vi "X calculator.vi"(9 "Blue":i16, 10 "Green":i16, 11 "Red":i16) -> (3 "X":dbl)   [LabVIEW 2014, in "AMS TS3472 Light Sensor.lvlib" / "AMS TCS3472.lvclass"]
uses:
  AMS TCS3472.lvclass
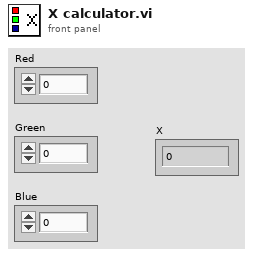
[diagram p1: front panel]
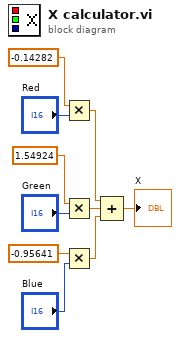
[diagram p0: block diagram]
diagram:
  n1 = Multiply(x=-0.14282, y="Red") -> (x*y=w7:dbl)
  n2 = Multiply(x=1.54924, y="Green") -> (x*y=w6:dbl)
  n3 = Multiply(x=-0.95641, y="Blue") -> (x*y=w5:dbl)
  n4 = Compound Arithmetic op=ADD(w7, w6, w5) -> (→"X":dbl)
